vi "Read Parent Hwnd.vi"(8 "error in (no error)":errorcluster, 11 "LV MDI in":refnum<class "LV MDI.lvclass">) -> (0 "error out":errorcluster, 2 "Parent Hwnd":i32, 3 "LV MDI out":refnum<class "LV MDI.lvclass">)   [LabVIEW 2019, in "LV MDI.lvclass"]
uses:
  LV MDI.lvclass
  LV MDI.lvclass/LV MDI.ctl
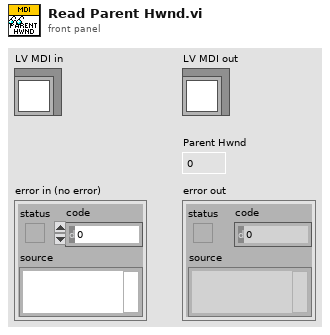
[diagram p1: front panel]
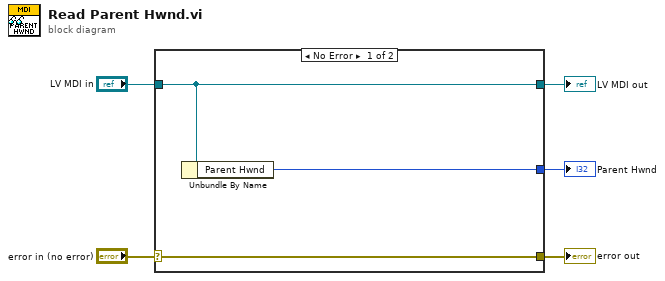
[diagram p0: block diagram]
diagram:
  n1 = case shown="No Error" "error in (no error)" {
    selector: "error in (no error)" -> [w8 w9]
    tunnel: [w8 w9] -> w4
    tunnel: [w7 w10] -> w2
    tunnel: "LV MDI in" -> [w7 w10]
    tunnel: [w6 _] -> w1
    frame No Error {
      n2 = Unbundle By Name(w7) -> ("Parent Hwnd"=w6:i32)
    }
    frame Error {
    }
  }
  "error out" <- w4
  "LV MDI out" <- w2
  "Parent Hwnd" <- w1
